vi "Save for Previous Version.vi"(8 "error in (no error)":errorcluster, 10 "LabVIEW Version":string, 11 "LabVIEW Class File in":refnum<class "LabVIEW Class File.lvclass">) -> (0 "error out":errorcluster, 1 "Errors":string, 2 "Warnings":string, 3 "LabVIEW Class File out":refnum<class "LabVIEW Class File.lvclass">)   [LabVIEW 2020, in "Save for Previous Version.lvlib" / "LabVIEW Class File.lvclass"]
uses:
  LabVIEW Class File.lvclass
  \\Mac\Home/JKI/GitHub/vipm-io/a-version-explorer-for-labview/experiments/save-for-previous-version/source/File/File.lvclass/File.lvclass
  File/File.lvclass/File.lvclass/File.ctl
  File/File.lvclass/Read Path.vi
  LabVIEW Class File.lvclass/LabVIEW Class File.ctl
  LabVIEW File/LabVIEW File.lvclass
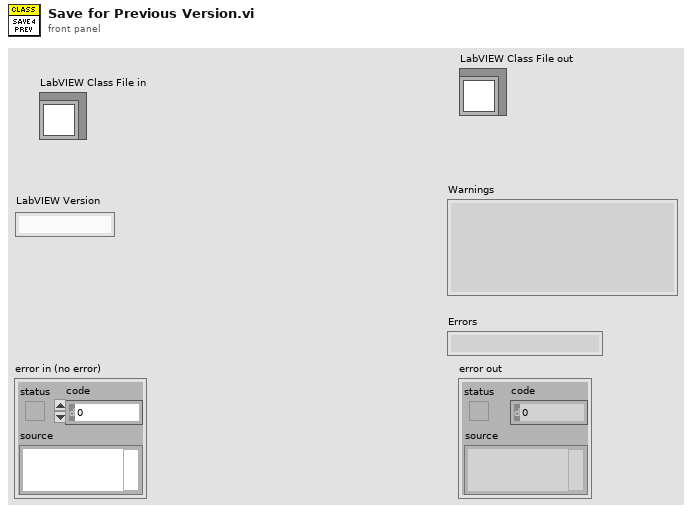
[diagram p1: front panel]
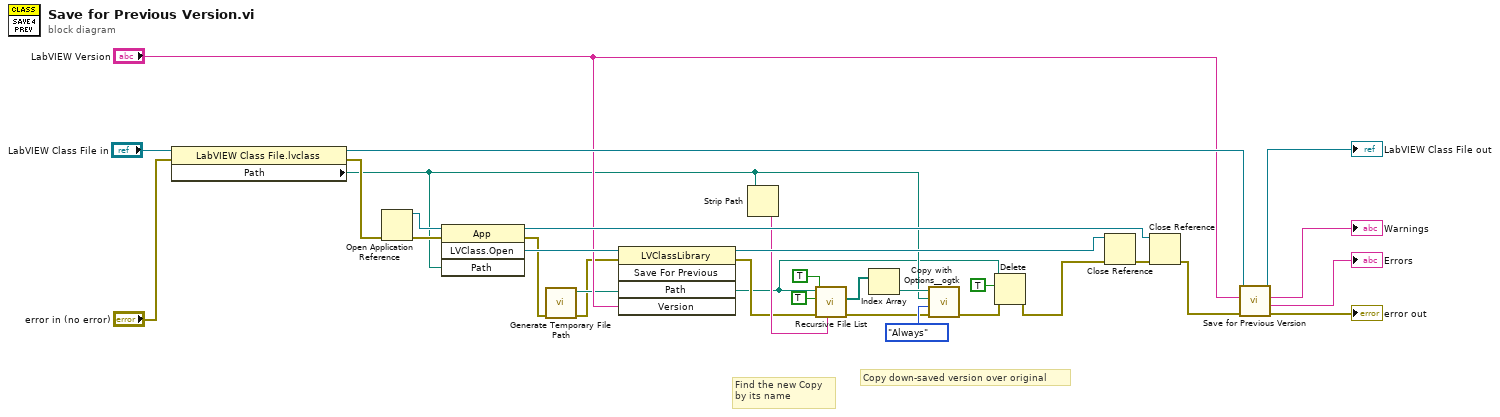
[diagram p0: block diagram]
diagram:
  # "Find the new Copy\nby its name"
  # "Copy down-saved version over original"
  n1 = property class="LabVIEW Class File.lvclass"(reference="LabVIEW Class File in", error in="error in (no error)") -> (reference out=w25:refnum<class "LabVIEW Class File.lvclass">, error out=w24:errorcluster, "Path"=w10:path)
  n2 = Open Application Reference(8:w24) -> (0:w31:errorcluster, 3:w30:refnum<vi>)  [unwired: 3 in]
  n3 = invoke class="App" method="LVClass.Open"(reference=w30, error in=w31, "Path"=w10) -> (reference out=w26:refnum<vi>, error out=w2:errorcluster, "LVClass.Open"=w29:refnum<vi>)  [unwired: 1 in, 1 out]
  n4 = call <vilib>:"Generate Temporary File Path.vi"("error in (no error)"=w2) -> ("error out"=w1:errorcluster, "Unique Temporary File Path"=w4:path)  [unwired: 9 in]
  n5 = invoke class="LVClassLibrary" method="Save For Previous"(reference=w29, error in=w1, "Path"=w4, "Version"="LabVIEW Version") -> (reference out=w28:refnum<vi>, error out=w7:errorcluster)  [unwired: 1 in, 3 out]
  n6 = Strip Path(path=w10) -> (name=w15:string)  [unwired: 1 out]
  n7 = call <vilib>:"Recursive File List.vi"("pattern"=w15, "error in (no error)"=w7, "Continue Recursing on Error? (F)"=TRUE, "Treat LLBs as Folders?"=TRUE, "Folder Path"=w4) -> ("error out"=w8:errorcluster, "All Files in Dir"=w12:path[])  [unwired: 2 in, 3 out]
  n8 = Index Array(array=w12) -> (element=w11:path)  [unwired: 1 in]
  n9 = call <userlib>:"Copy with Options__ogtk.vi"("error in (no error)"=w8, "Replace Mode (Never)"=enum16{"Never", "Always", "If Newer"}."Always", "target path"=w10, "source path"=w11) -> ("error out"=w6:errorcluster)  [unwired: 6 in, 1 out]
  n10 = Delete(path (use dialog)=w4, entire hierarchy (F)=TRUE, error in=w6) -> (error out=w5:errorcluster)  [unwired: 2 in, 2 out]
  n11 = Close Reference(reference=w28, error in (no error)=w5) -> (error out=w27:errorcluster)
  n12 = Close Reference(reference=w26, error in (no error)=w27) -> (error out=w23:errorcluster)
  n13 = call-parent "Save for Previous Version.vi"("error in (no error)"=w23, "LabVIEW Version"="LabVIEW Version", "LabVIEW File in"=w25) -> ("error out"=→"error out":errorcluster, "Errors"=→"Errors":string, "Warnings"=→"Warnings":string, "LabVIEW File out"=→"LabVIEW Class File out":refnum<class "LabVIEW Class File.lvclass">)  [unwired: 5 in]
